vi "Configure User Margin.vi"(8 "error in (no error)":errorcluster, 9 "User Margin (0)":dbl format="%^.3e", 10 "Instance (1)":i32=1, 11 "VISA resource name":refnum<visa-resource-name>) -> (0 "error out":errorcluster, 3 "VISA resource name out":refnum<visa-resource-name>)   [LabVIEW 2015, in "Rohde&Schwarz CMP LR WPAN Measurement.lvlib"]
doc: "Sets the margin that the measurement adds to the expected nominal power to determine the reference level. The reference level minus the external input attenuation must be within the power range of the selected input connector; refer to the data sheet.\n\nAttribute:\nRSCMPLRWM_ATTR_USER_MARGIN\n\nRemote-control command:\nCONFigure:WPAN:MEAS<i>:RFSettings:UMARgin"
uses:
  <instrlib>/Rohde&Schwarz CMP LR WPAN Measurement/Rohde&Schwarz CMP LR WPAN Measurement.lvlib
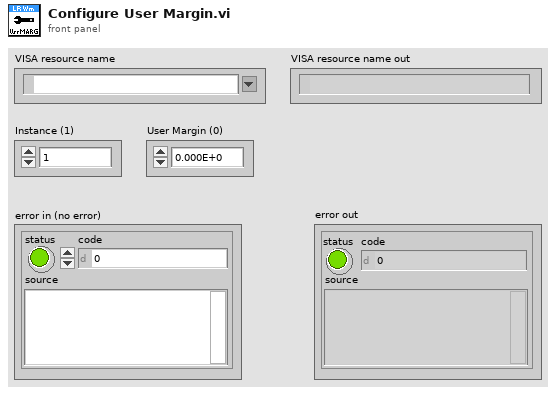
[diagram p1: front panel]
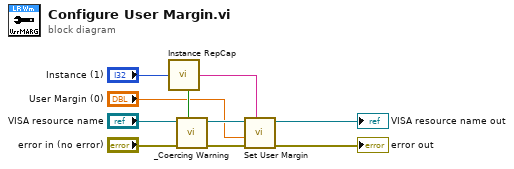
[diagram p0: block diagram]
diagram:
  n1 = call <instrlib>:"Instance RepCap.vi"("Instance In"="Instance (1)") -> ("In Range?"=w8:bool, "RepCap Identifier Out"=w7:string)  [unwired: 1 in]
  n2 = call <instrlib>:"_Coercing Warning.vi"("In Range?"=w8, "error in (no error)"="error in (no error)", "VISA resource name"="VISA resource name") -> ("error out"=w4:errorcluster, "VISA resource name out"=w3:refnum<visa-resource-name>)  [unwired: 7 in]
  n3 = call "Set User Margin"("Repeated Capabilities"=w7, "error in (no error)"=w4, "User Margin (0.0)"="User Margin (0)", "instrument handle"=w3) -> ("error out"=→"error out":errorcluster, "instrument handle out"=→"VISA resource name out":refnum<visa-resource-name>)  [unwired: 6 in]
